vi "Flatten.vi"(8 "error in":errorcluster, 9 "Data":T1) -> (0 "error out":errorcluster, 2 "Buffer":u8[](array[numeric]) format="%.0x")   [LabVIEW 2020, in "Discovery.lvlib"]
uses:
  Discovery.lvlib
  Data.ctl
  Service/Data.ctl
  ServiceType/Enumeration.ctl
  <vilib>/IlluminatedG/IG Protoc/LV-Proto/Wire Encode Tag.vi
  <vilib>/IlluminatedG/IG Protoc/LV-Proto/Encode bytes.vi
  <vilib>/IlluminatedG/IG Protoc/LV-Proto/Wire Encode Varint I32.vi
  <vilib>/IlluminatedG/IG Protoc/LV-Proto/Encode LEN.vi
  <vilib>/IlluminatedG/IG Protoc/LV-Proto/LV-Proto.lvlib
  Service/Service.lvlib
  ServiceType/ServiceType.lvlib
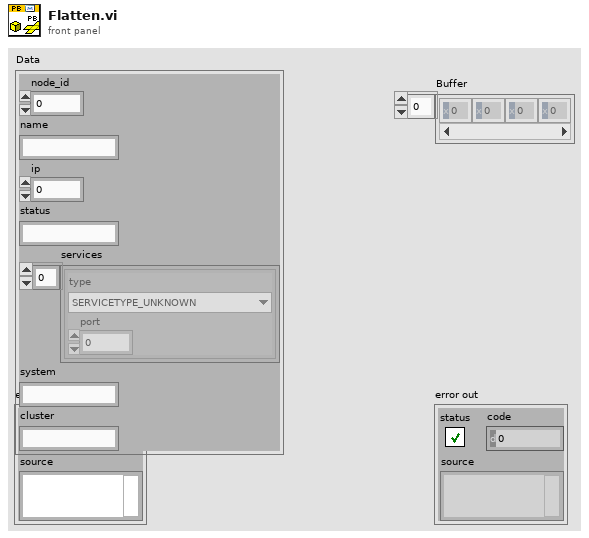
[diagram p1: front panel]
types:
  T1 = typedef "Discovery.lvlib/Data.ctl" = cluster{"node_id":u32, "name":string, "ip":u32, "status":string, "services":T2[], "system":string, "cluster":string}
  T2 = typedef "Service.lvlib/Data.ctl" = cluster{"type":T3, "port":i32}
  T3 = typedef "ServiceType.lvlib/Enumeration.ctl" = enum16{"SERVICETYPE_UNKNOWN", "SERVICETYPE_TCPSERVER", "SERVICETYPE_HTTPSERVER"}
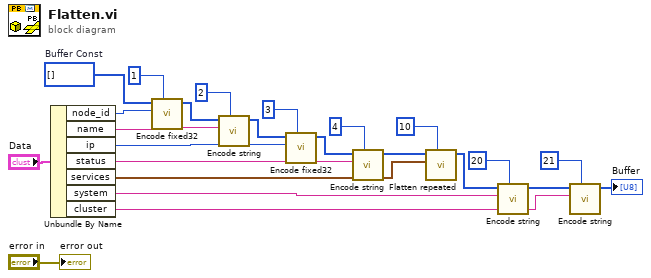
[diagram p0: block diagram]
diagram:
  w22 = u8[] []  # Buffer Const
  n1 = Unbundle By Name("Data") -> ("node_id"=w20:u32, "name"=w17:string, "ip"=w14:u32, "status"=w11:string, "services"=w9:T2[], "system"=w5:string, "cluster"=w2:string)
  n2 = call <vilib>:"Encode fixed32.vi"("Field Number"=1, "fixed32"=w20, "Buffer in"=w22) -> ("Buffer"=w19:u8[])  [unwired: 8 in]
  n3 = call <vilib>:"Encode string.vi"("Field Number"=2, "string"=w17, "Buffer in"=w19) -> ("Buffer"=w16:u8[])  [unwired: 8 in]
  n4 = call <vilib>:"Encode fixed32.vi"("Field Number"=3, "fixed32"=w14, "Buffer in"=w16) -> ("Buffer"=w13:u8[])  [unwired: 8 in]
  n5 = call <vilib>:"Encode string.vi"("Field Number"=4, "string"=w11, "Buffer in"=w13) -> ("Buffer"=w10:u8[])  [unwired: 8 in]
  n6 = call "Flatten repeated.vi"("Field Number"=10, "Data"=w9, "Buffer in"=w10) -> ("Buffer"=w7:u8[])  [unwired: 8 in]
  n7 = call <vilib>:"Encode string.vi"("Field Number"=20, "string"=w5, "Buffer in"=w7) -> ("Buffer"=w4:u8[])  [unwired: 8 in]
  n8 = call <vilib>:"Encode string.vi"("Field Number"=21, "string"=w2, "Buffer in"=w4) -> ("Buffer"=→"Buffer":u8[])  [unwired: 8 in]
  "error out" <- "error in"
